vi "Julian_quiz1.vi"() -> ()   [LabVIEW 2020]
uses:
  Control 1.ctl
panel:
  in  "Go to state 0":bool
  in  "stop":bool
  out "State #":dbl
  out "Current State":dbl
  out "# Go to State 0":dbl
  out "Iteration #":dbl
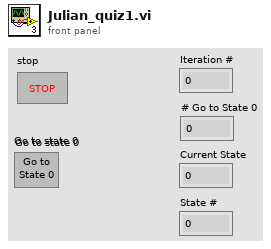
[diagram p1: front panel]
types:
  T1 = typedef "Control 1.ctl" = enum16{"State 0", "State 1", "State 2", "State 3", "State 4", "State 5"}
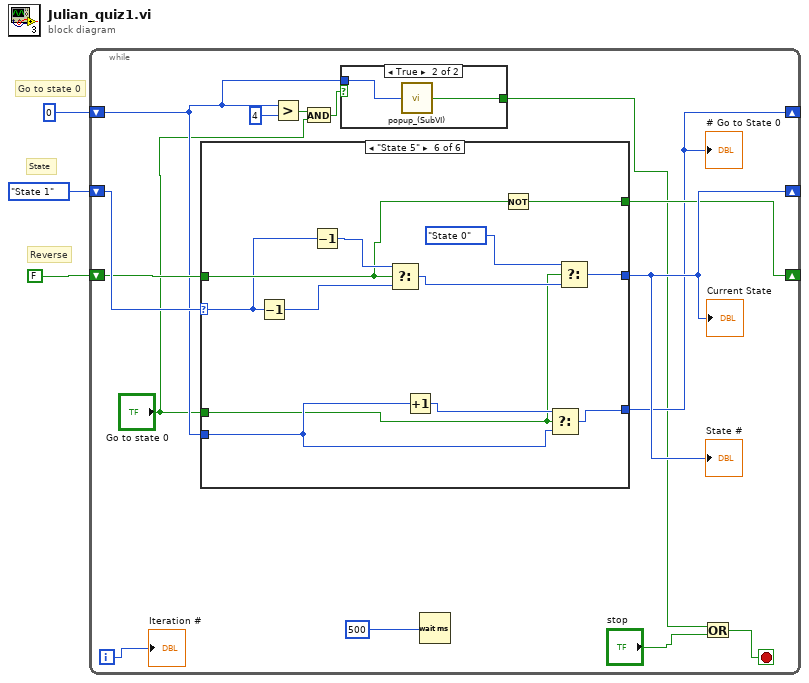
[diagram p0: block diagram]
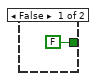
[diagram p2: hidden frame]
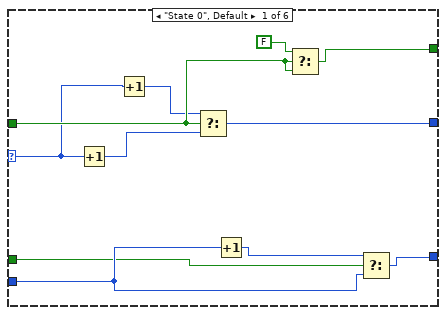
[diagram p3: hidden frame]
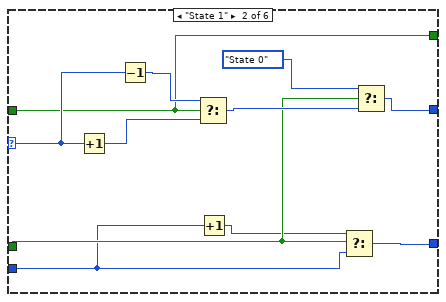
[diagram p4: hidden frame]
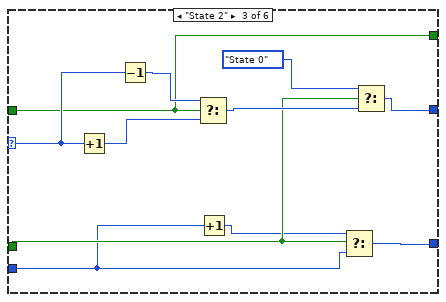
[diagram p5: hidden frame]
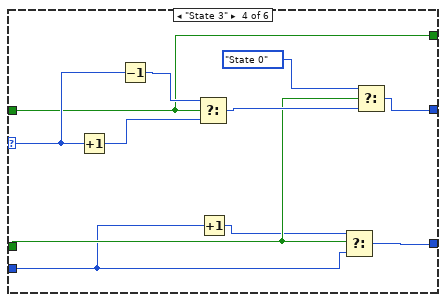
[diagram p6: hidden frame]
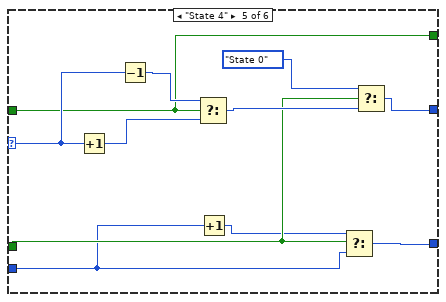
[diagram p7: hidden frame]
diagram:
  # "Reverse"
  # "State"
  # "Go to state 0"
  n1 = while {
    shift-right: [w12] -> _
    shift-left: 0 -> [w10]
    shift-right: [w14] -> _
    shift-left: Control_1."State 1" -> [w16]
    shift-right: [w13] -> _
    shift-left: FALSE -> [w15]
    i -> [w18]
    stop <- w7 stop-if-true
    n2 = case shown="\"State 5\"" w16 {
      selector: w16 -> [w27 w41 w52 w63 w74 w85]
      tunnel: w15 -> [w30 w40 w51 w62 w73 w87]
      tunnel: [w31 w37 w48 w59 w70 w79] -> w14
      tunnel: [w28 w40 w51 w62 w73 w86] -> w13
      tunnel: "Go to state 0" -> [w23 w36 w47 w58 w69 w77]
      tunnel: w10 -> [w24 w33 w44 w55 w66 w82]
      tunnel: [w22 w35 w46 w57 w68 w81] -> w12
      frame "State 0", Default {
        n3 = Increment(x=w27) -> (x+1=w32:T1)
        n4 = Increment(x=w27) -> (x+1=w26:T1)
        n5 = Select(t=w26, s=w30, f=w32) -> (s? t:f=w31:T1)
        n6 = Increment(x=w24) -> (x+1=w25:i32)
        n7 = Select(t=FALSE, s=w30, f=w30) -> (s? t:f=w28:bool)
        n8 = Select(t=w25, s=w23, f=w24) -> (s? t:f=w22:i32)
      }
      frame "State 1" {
        n9 = Increment(x=w41) -> (x+1=w43:T1)
        n10 = Decrement(x=w41) -> (x-1=w42:T1)
        n11 = Select(t=w42, s=w40, f=w43) -> (s? t:f=w39:T1)
        n12 = Increment(x=w33) -> (x+1=w34:i32)
        n13 = Select(t=w34, s=w36, f=w33) -> (s? t:f=w35:i32)
        n14 = Select(t=Control_1."State 0", s=w36, f=w39) -> (s? t:f=w37:T1)
      }
      frame "State 2" {
        n15 = Increment(x=w52) -> (x+1=w54:T1)
        n16 = Decrement(x=w52) -> (x-1=w53:T1)
        n17 = Select(t=w53, s=w51, f=w54) -> (s? t:f=w50:T1)
        n18 = Increment(x=w44) -> (x+1=w45:i32)
        n19 = Select(t=w45, s=w47, f=w44) -> (s? t:f=w46:i32)
        n20 = Select(t=Control_1."State 0", s=w47, f=w50) -> (s? t:f=w48:T1)
      }
      frame "State 3" {
        n21 = Increment(x=w63) -> (x+1=w65:T1)
        n22 = Decrement(x=w63) -> (x-1=w64:T1)
        n23 = Select(t=w64, s=w62, f=w65) -> (s? t:f=w61:T1)
        n24 = Increment(x=w55) -> (x+1=w56:i32)
        n25 = Select(t=w56, s=w58, f=w55) -> (s? t:f=w57:i32)
        n26 = Select(t=Control_1."State 0", s=w58, f=w61) -> (s? t:f=w59:T1)
      }
      frame "State 4" {
        n27 = Increment(x=w74) -> (x+1=w76:T1)
        n28 = Decrement(x=w74) -> (x-1=w75:T1)
        n29 = Select(t=w75, s=w73, f=w76) -> (s? t:f=w72:T1)
        n30 = Increment(x=w66) -> (x+1=w67:i32)
        n31 = Select(t=w67, s=w69, f=w66) -> (s? t:f=w68:i32)
        n32 = Select(t=Control_1."State 0", s=w69, f=w72) -> (s? t:f=w70:T1)
      }
      frame "State 5" {
        n33 = Decrement(x=w85) -> (x-1=w84:T1)
        n34 = Decrement(x=w85) -> (x-1=w88:T1)
        n35 = Select(t=w88, s=w87, f=w84) -> (s? t:f=w78:T1)
        n36 = Increment(x=w82) -> (x+1=w83:i32)
        n37 = Not(x=w87) -> (.not. x?=w86:bool)
        n38 = Select(t=w83, s=w77, f=w82) -> (s? t:f=w81:i32)
        n39 = Select(t=Control_1."State 0", s=w77, f=w78) -> (s? t:f=w79:T1)
      }
    }
    "# Go to State 0" <- w12
    "Current State" <- w14
    "State #" <- w14
    n40 = Greater?(x=w10, y=4) -> (0:w5:bool)
    n41 = And(x=w5, y="Go to state 0") -> (x .and. y?=w6:bool)
    n42 = case shown="True" w6 {
      tunnel: w10 -> [_ w21]
      tunnel: [FALSE ("Boolean") w20] -> w8
      frame False {
      }
      frame True {
        n43 = call "popup_(SubVI).vi"("X"=w21) -> ("Boolean"=w20:bool)
      }
    }
    n44 = Wait (ms)(milliseconds to wait=500) -> ()  [unwired: 1 out]
    n45 = Or(x=w8, y="stop") -> (x .or. y?=w7:bool)
    "Iteration #" <- w18
  }
